vi "Item_OnPopupMenu.vi"(11 "Item Ref":T1) -> ()   [LabVIEW 2020, in "Negentropic IDE.lvlib"]
uses:
  Negentropic IDE.lvlib
  <resource>/Framework/Providers/API/ItemRef.ctl
  <resource>/Framework/Providers/API/mxLvMenuItem.ctl
  <vilib>/Utility/config.llb/Read Key (String).vi
  <vilib>/Utility/config.llb/NI_LVConfig.lvlib
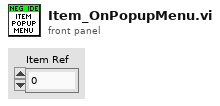
[diagram p1: front panel]
types:
  T1 = typedef "ItemRef.ctl" = u64
  T2 = typedef "mxLvMenuItem.ctl" = cluster{"Menu Name":string, "Description":string, "Icon File Name":path, "Menu Tag":string, "Enabled":bool, "Checked":bool, "Separator":bool, "Batchable":bool, "Weight":i32, "Batch Mode (Ignored if Not Batchable)":enum32{"Show If All Items Support Command", "Show If Any Items Support Command"}, "Menu Location":enum32{"<None>", "Project", "Project / Build Specifications", "Tools", "Tools / Source Control", "Tools / Real-Time Module", "Help"}, "Exclude From Getting Started Window Menu":bool}
  T3 = typedef "NI_LVConfig.lvlib/Config Data RefNum.ctl" = refnum<k1>
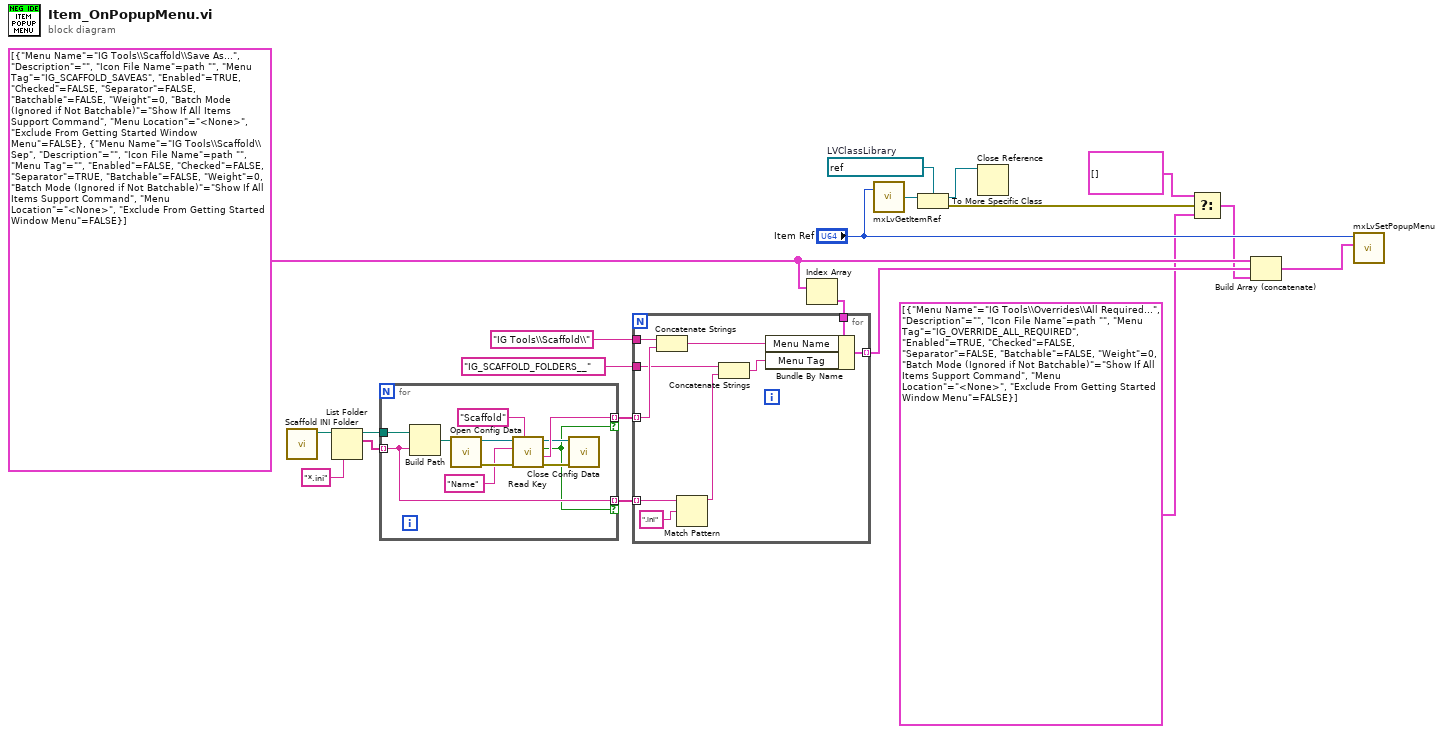
[diagram p0: block diagram]
diagram:
  w7 = refnum<vi> refnum  # LVClassLibrary
  w14 = T2[] [{"Menu Name"="IG Tools\\Scaffold\\Save As...", "Description"="", "Icon File Name"=path "", "Menu Tag"="IG_SCAFFOLD_SAVEAS", "Enabled"=TRUE, "Checked"=FALSE, "Separator"=FALSE, "Batchable"=FALSE, "Weight"=0, "Batch Mode (Ignored if Not Batchable)"=enum."Show If All Items Support Command", "Menu Location"=enum."<None>", "Exclude From Getting Started Window Menu"=FALSE}, {"Menu Name"="IG Tools\\Scaffold\\Sep", "Description"="", "Icon File Name"=path "", "Menu Tag"="", "Enabled"=FALSE, "Checked"=FALSE, "Separator"=TRUE, "Batchable"=FALSE, "Weight"=0, "Batch Mode (Ignored if Not Batchable)"=enum."Show If All Items Support Command", "Menu Location"=enum."<None>", "Exclude From Getting Started Window Menu"=FALSE}] ("Popup Menu Items")
  n1 = call "Scaffold INI Folder.vi"() -> ("Scaffold INI Folder"=w20:path)  [unwired: 10 in, 1 out]
  n2 = List Folder(path=w20, pattern="*.ini") -> (path out=w18:path, filenames=w17:string[])  [unwired: 2 in, 2 out]
  n3 = for {
    tunnel: w18 -> [w31]
    tunnel: w17 -> [w22] mode=indexing
    tunnel: [w25] -> w16 mode=indexing if=w21
    tunnel: [w22] -> w12 mode=indexing if=w21
    n4 = Build Path(base path=w31, name or relative path=w22) -> (appended path=w30:path)
    n5 = call <vilib>:"Open Config Data.vi"("configuration file path"=w30) -> ("error out"=w28:errorcluster, "refnum"=w29:T3)  [unwired: 8 in, 1 out]
    n6 = call-poly <vilib>:"Read Key.vi"("section"="Scaffold", "error in (no error)"=w28, "key"="Name", "refnum"=w29) -> ("error out"=w23:errorcluster, "value"=w25:string, "found?"=w21:bool, "refnum out"=w24:T3)  [unwired: 4 in]
    n7 = call <vilib>:"Close Config Data.vi"("error in (no error)"=w23, "refnum"=w24) -> ()  [unwired: 8 in, 2 out]
  }
  n8 = Index Array(array=w14) -> (element=w13:T2)  [unwired: 1 in]
  n9 = for {
    tunnel: w16 -> [w40] mode=indexing
    tunnel: "IG Tools\\Scaffold\\" -> [w41]
    tunnel: w13 -> [w39]
    tunnel: w12 -> [w37] mode=indexing
    tunnel: "IG_SCAFFOLD_FOLDERS__" -> [w35]
    tunnel: [w32] -> w9 mode=indexing
    n10 = Concatenate Strings(w41, w40) -> (w38:string)
    n11 = Match Pattern(string=w37, regular expression=".ini") -> (before substring=w34:string)  [unwired: 1 in, 3 out]
    n12 = Concatenate Strings(w35, w34) -> (w33:string)
    n13 = Bundle By Name(cluster=w39, "Menu Name"=w38, "Menu Tag"=w33) -> (w32:T2)
  }
  n14 = call <resource>:"mxLvGetItemRef.vi"("Item"="Item Ref") -> ("Item Refnum"=w8:refnum<vi>)  [unwired: 1 in, 2 out]
  n15 = To More Specific Class(target class=w7, reference=w8) -> (specific class reference=w1:refnum<vi>, error out=w4:errorcluster)  [unwired: 1 in]
  n16 = Close Reference(reference=w1) -> ()  [unwired: 1 in, 1 out]
  n17 = Select(t=T2[] [], s=w4, f=T2[] [{"Menu Name"="IG Tools\\Overrides\\All Required...", "Description"="", "Icon File Name"=path "", "Menu Tag"="IG_OVERRIDE_ALL_REQUIRED", "Enabled"=TRUE, "Checked"=FALSE, "Separator"=FALSE, "Batchable"=FALSE, "Weight"=0, "Batch Mode (Ignored if Not Batchable)"=enum."Show If All Items Support Command", "Menu Location"=enum."<None>", "Exclude From Getting Started Window Menu"=FALSE}] ("Popup Menu Items")) -> (s? t:f=w2:T2[])
  n18 = Build Array (concatenate)(w14, w9, w2) -> (w10:T2[])
  n19 = call <resource>:"mxLvSetPopupMenu.vi"("Popup Menu Items"=w10, "Item"="Item Ref") -> ()  [unwired: 8 in, 2 out]
